vi "New JSON Array (NULL).vi"(8 "error in (no error)":errorcluster) -> (0 "error out":errorcluster, 3 "JSON Array out":refnum<class "JSON Array.lvclass">)   [LabVIEW 2017, in "LVJSON.lvlib" / "JSON Array.lvclass"]
uses:
  JSON Array.lvclass
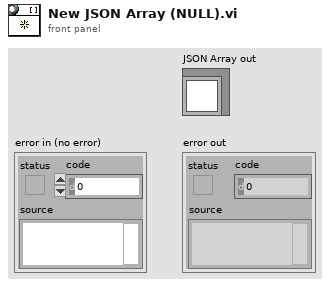
[diagram p1: front panel]
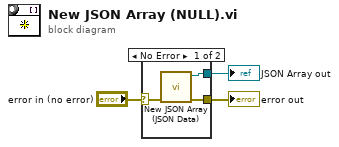
[diagram p0: block diagram]
diagram:
  n1 = case shown="No Error" "error in (no error)" {
    selector: "error in (no error)" -> [w5 w7]
    tunnel: [w4 w7] -> w2
    tunnel: [w6 _] -> w1
    frame No Error {
      n2 = call "New JSON Array (JSON Data).vi"("error in (no error)"=w5) -> ("error out"=w4:errorcluster, "JSON Array out"=w6:refnum<class "JSON Array.lvclass">)  [unwired: 9 in]
    }
    frame Error {
    }
  }
  "error out" <- w2
  "JSON Array out" <- w1
